vi "z internal subscriber check.vi"(8 "error in (no error)":errorcluster, 11 "this_":cluster{}) -> (0 "error out":errorcluster, 3 "function return":bool)   [LabVIEW 2021, in "zenohc.lvlib"]
doc: "ZENOHC_API bool z_internal_subscriber_check(const struct z_owned_subscriber_t *this_);"
uses:
  zenohc.lvlib
  zenohc.dll
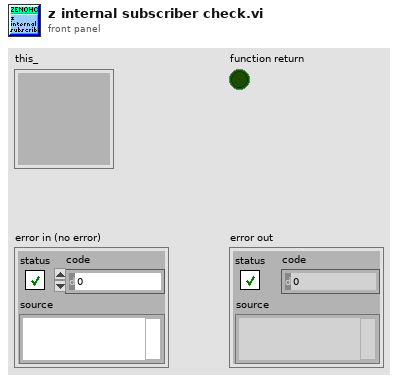
[diagram p1: front panel]
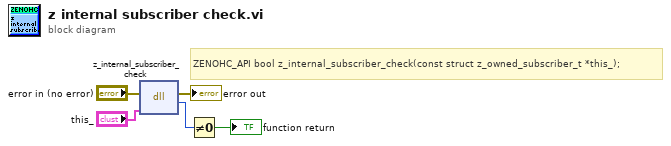
[diagram p0: block diagram]
diagram:
  # "ZENOHC_API bool z_internal_subscriber_check(const struct z_owned_subscriber_t *this_);"
  n1 = dll-call lib="D:/dev/zenoh_labview/zenohc/zenohc.*" fn="z_internal_subscriber_check"(error in="error in (no error)", "this_"="this_") -> (error out=→"error out":errorcluster, w4:u8)  [unwired: 3 in, 1 out]
  n2 = Not Equal To 0?(x=w4) -> (x != 0?=→"function return":bool)
